vi "Utility_GenerateInstructions.vi"() -> (1 "size(s)":i32, 3 "Instruction":cluster{"RightW":dbl, "LeftW":dbl}[](array[cluster]))   [LabVIEW 2010]
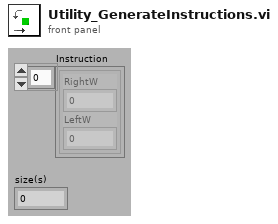
[diagram p1: front panel]
types:
  T1 = cluster{"number: 0 to 1":dbl, cluster{dbl, dbl}}[]
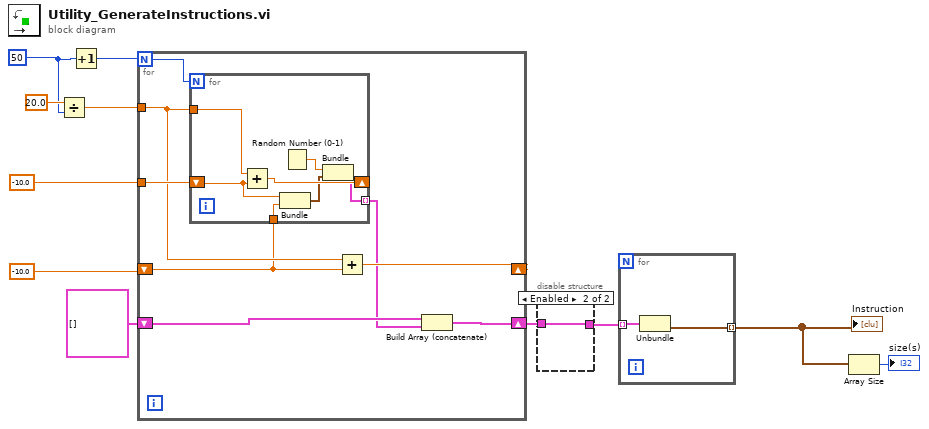
[diagram p0: block diagram]
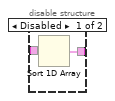
[diagram p2: hidden frame]
diagram:
  w7 = 50
  n1 = Divide(x=20.0, y=w7) -> (x/y=w8:dbl)
  n2 = Increment(x=w7) -> (x+1=w6:i32)
  n3 = for {
    N: w6 -> [w18]
    tunnel: -10.0 -> [w19]
    tunnel: w8 -> [w17]
    shift-right: [w16] -> _
    shift-left: -10.0 -> [w13]
    shift-right: [w14] -> w2
    shift-left: T1 [] -> [w15]
    n4 = for {
      N: w18 -> [_]
      shift-right: [w25] -> _
      shift-left: w19 -> [w24]
      tunnel: w17 -> [w26]
      tunnel: w13 -> [w23]
      tunnel: [w20] -> w12 mode=indexing
      n5 = Add(x=w26, y=w24) -> (x+y=w25:dbl)
      n6 = Bundle(w24, w23) -> (w21:cluster{dbl, dbl})  [unwired: 1 in]
      n7 = Random Number (0-1)() -> (number: 0 to 1=w22:dbl)
      n8 = Bundle("number: 0 to 1"=w22, w21) -> (w20:cluster{"number: 0 to 1":dbl, cluster{dbl, dbl}})  [unwired: 1 in]
    }
    n9 = Add(x=w17, y=w13) -> (x+y=w16:dbl)
    n10 = Build Array (concatenate)(w15, w12) -> (w14:T1)
  }
  n11 = disable-structure shown="Enabled" {
    disable-tunnel: [w28 w29] -> w4
    disable-tunnel: w2 -> [w27 w29]
    frame Disabled {
      n12 = Sort 1D Array(array=w27) -> (sorted array=w28:T1)
    }
    frame Enabled {
    }
  }
  n13 = for {
    tunnel: w4 -> [w31] mode=indexing
    tunnel: [w30] -> w1 mode=indexing
    n14 = Unbundle(w31) -> (w30:cluster{dbl, dbl})  [unwired: 1 out]
  }
  "Instruction" <- w1
  n15 = Array Size(array=w1) -> (size(s)=→"size(s)":i32)
